vi "Encode Signature.vi"(7 "Signature Method":T1=enum."HMAC-SHA1", 8 "error in (no error)":errorcluster, 9 "Signature Base string":string, 10 "consumer secret":string, 11 "access token secret":string) -> (0 "error out":errorcluster, 2 "Encoded Signature":string)   [LabVIEW 2011, in "i3-oauth.lvlib"]
uses:
  i3-oauth.lvlib
  Controls/Signature Method.ctl
  i3-external-encryption/labviewencryption/hash-types.ctl
  i3-external-encryption/i3-external-encryption.lvlib
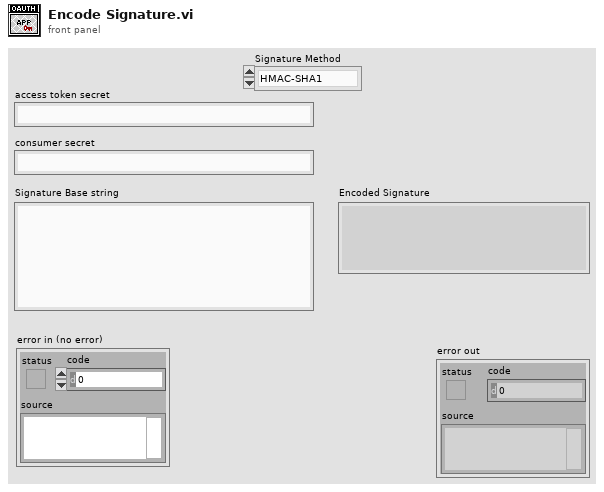
[diagram p1: front panel]
types:
  T1 = typedef "i3-oauth.lvlib/Signature Method.ctl" = enum16{"HMAC-MD5", "HMAC-SHA1", "HMAC-SHA224", "HMAC-SHA256", "HMAC-SHA384", "HMAC-SHA512"}
  T2 = typedef "i3-external-encryption.lvlib/hash-types.ctl" = enum16{"MD5", "SHA-1", "SHA-224", "SHA-256", "SHA-384", "SHA-512"}
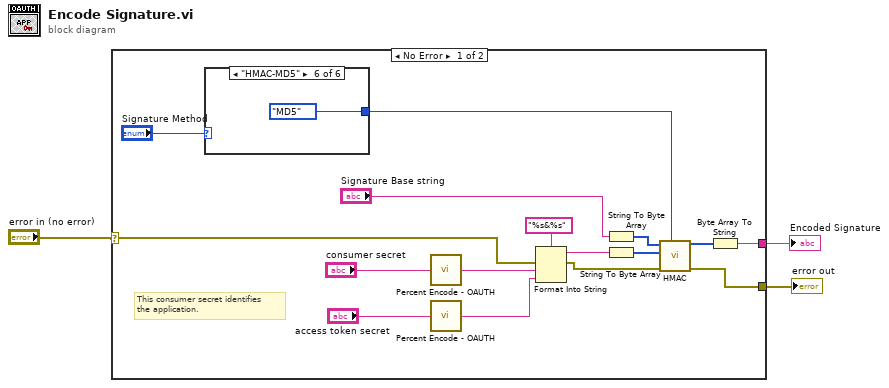
[diagram p0: block diagram]
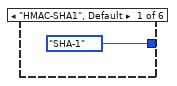
[diagram p2: hidden frame]
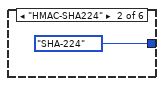
[diagram p3: hidden frame]
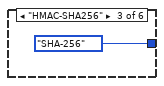
[diagram p4: hidden frame]
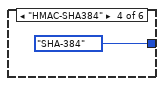
[diagram p5: hidden frame]
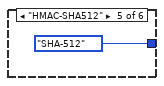
[diagram p6: hidden frame]
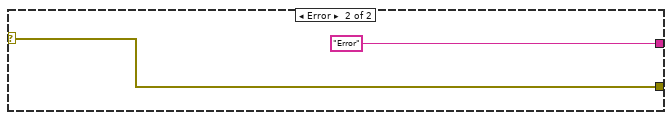
[diagram p7: hidden frame]
diagram:
  n1 = case shown="No Error" "error in (no error)" {
    selector: "error in (no error)" -> [w7 w27]
    tunnel: [w10 "Error"] -> w3
    tunnel: [w8 w27] -> w2
    frame No Error {
      # "This consumer secret identifies\nthe application."
      n2 = case shown="\"HMAC-MD5\"" "Signature Method" {
        tunnel: [hash-types."SHA-1" ("HASH-method 2") hash-types."SHA-224" ("HASH-method 2") hash-types."SHA-256" ("HASH-method 2") hash-types."SHA-384" ("HASH-method 2") hash-types."SHA-512" ("HASH-method 2") hash-types."MD5" ("HASH-method 2")] -> w5
        frame "HMAC-SHA1", Default {
        }
        frame "HMAC-SHA224" {
        }
        frame "HMAC-SHA256" {
        }
        frame "HMAC-SHA384" {
        }
        frame "HMAC-SHA512" {
        }
        frame "HMAC-MD5" {
        }
      }
      n3 = call "Percent Encode - OAUTH.vi"("unescaped string in"="consumer secret") -> ("escaped string out"=w18:string)
      n4 = call "Percent Encode - OAUTH.vi"("unescaped string in"="access token secret") -> ("escaped string out"=w17:string)
      n5 = Format Into String(format string="%s&%s", error in=w7, w18, w17) -> (resulting string=w11:string, error out=w9:errorcluster)  [unwired: 1 in]
      n6 = String To Byte Array(string="Signature Base string") -> (unsigned byte array=w15:u8[])
      n7 = String To Byte Array(string=w11) -> (unsigned byte array=w14:u8[])
      n8 = call "HMAC.vi"("HASH-method"=w5, "error in (no error)"=w9, "Key"=w14, "Message"=w15) -> ("error out"=w8:errorcluster, "HMAC digest"=w13:u8[])  [unwired: 5 in, 1 out]
      n9 = Byte Array To String(unsigned byte array=w13) -> (string=w10:string)
    }
    frame Error {
    }
  }
  "error out" <- w2
  "Encoded Signature" <- w3
